vi "Info.vi"() -> (0 "error out":errorcluster, 2 "LibraryName":string, 3 "VI Name":string)   [LabVIEW 2011]
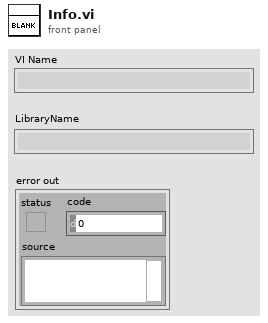
[diagram p1: front panel]
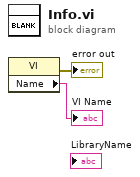
[diagram p0: block diagram]
diagram:
  n1 = property class="VI"() -> (error out=→"error out":errorcluster, "Name"=→"VI Name":string)  [unwired: 2 in, 1 out]
